vi "InputDialog.vi"(7 "Title":string, 8 "error in (no error)":errorcluster, 9 "Ctl Refnum":refnum<vi>, 11 "Name":string) -> (0 "error out":errorcluster, 1 "OK":bool, 3 "Name Out":string)   [LabVIEW 2015]
panel:
  in  "Cancel":bool
  in  "OK2":bool
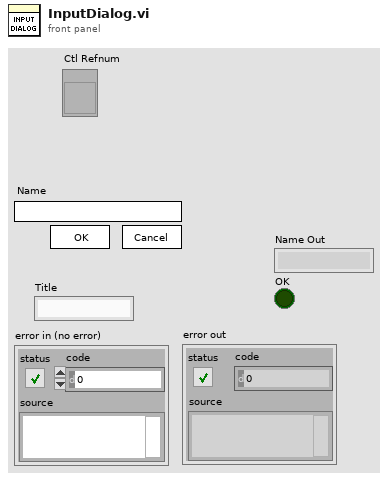
[diagram p1: front panel]
types:
  T1 = typedef "LVPositionTypeDef.ctl" = cluster{"Left":i32, "Top":i32}
  T2 = typedef "LVRectTypeDef.ctl" = cluster{"Left":i16, "Top":i16, "Right":i16, "Bottom":i16}
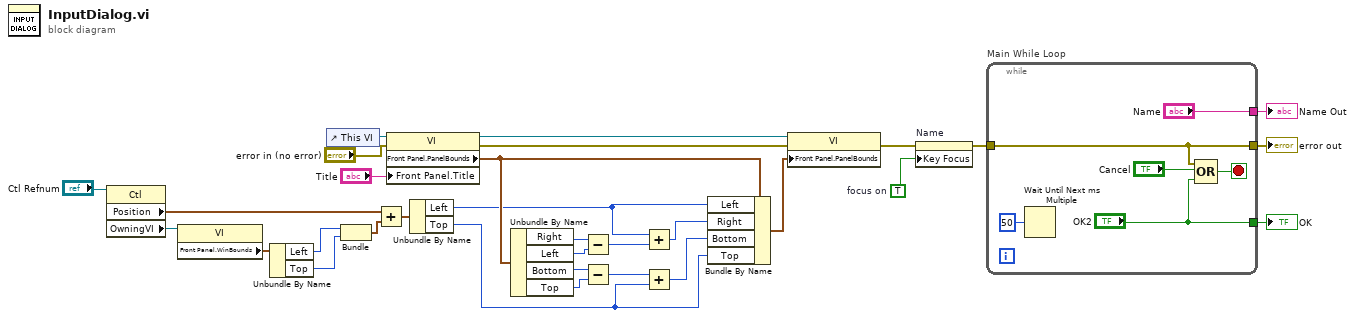
[diagram p0: block diagram]
diagram:
  w28 = TRUE  # focus on
  n1 = property on="Property Node" class="Ctl"(reference="Ctl Refnum") -> ("Position"=w3:T1, "OwningVI"=w8:refnum<vi>)  [unwired: 1 in, 2 out]
  n2 = property class="VI"(reference=w8) -> ("Front Panel.WinBounds"=w7:T2)  [unwired: 1 in, 2 out]
  n3 = Unbundle By Name(w7) -> ("Left"=w6:i16, "Top"=w5:i16)
  n4 = control-ref of="This VI"() -> (w27:refnum<vi>)
  n5 = Bundle("Left"=w6, "Top"=w5) -> (w4:cluster{"Left":i16, "Top":i16})  [unwired: 1 in]
  n6 = Add(x=w3, y=w4) -> (x+y=w1:T1)
  n7 = property class="VI"(reference=w27, error in="error in (no error)", "Front Panel.Title"="Title") -> (reference out=w24:refnum<vi>, error out=w23:errorcluster, "Front Panel.PanelBounds"=w15:T2)
  n8 = Unbundle By Name(w1) -> ("Left"=w13:i32, "Top"=w14:i32)
  n9 = Unbundle By Name(w15) -> ("Right"=w26:i16, "Left"=w17:i16, "Bottom"=w25:i16, "Top"=w16:i16)
  n10 = Subtract(x=w26, y=w17) -> (x-y=w22:i16)
  n11 = Subtract(x=w25, y=w16) -> (x-y=w21:i16)
  n12 = Add(x=w13, y=w22) -> (x+y=w20:i32)
  n13 = Add(x=w21, y=w14) -> (x+y=w19:i32)
  n14 = Bundle By Name(cluster=w15, "Left"=w13, "Right"=w20, "Bottom"=w19, "Top"=w14) -> (w18:T2)
  n15 = property class="VI"(reference=w24, error in=w23, "Front Panel.PanelBounds"=w18) -> (error out=w9:errorcluster)  [unwired: 1 out]
  n16 = property on="Name" class="Str"(error in=w9, "Key Focus"=w28) -> (error out=w12:errorcluster)  [unwired: 1 in, 1 out]
  n17 = while "Main While Loop" {
    tunnel: ["OK2"] -> w29
    tunnel: w12 -> [w35]
    tunnel: [w35] -> w31
    tunnel: ["Name"] -> w30
    stop <- w36 stop-if-true
    n18 = Wait Until Next ms Multiple(millisecond multiple=u32 50) -> ()  [unwired: 1 out]
    n19 = Compound Arithmetic op=OR(w35, "Cancel", "OK2") -> (w36:bool)
  }
  "error out" <- w31
  "Name Out" <- w30
  "OK" <- w29
